vi "OpenEthConnection.vi"(10 "Port":u16=80, 11 "IP address":string="192.168.1.150") -> (0 "error out":errorcluster, 3 "connection ID out":refnum<k5>, 4 "Answer":string="\n\r\n")   [LabVIEW 2015, in "VIPM2.lvlib"]
uses:
  VIPM2.lvlib
panel:
  # "Open Ethernet connection"
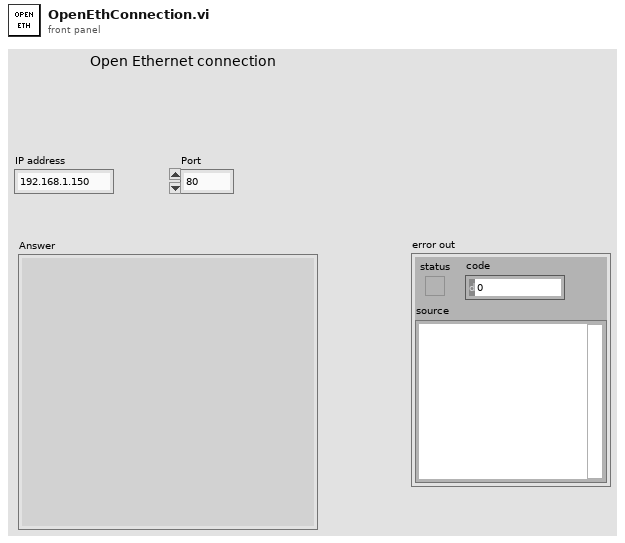
[diagram p1: front panel]
types:
  T1 = enum16{"Standard", "Buffered", "CRLF", "Immediate"}
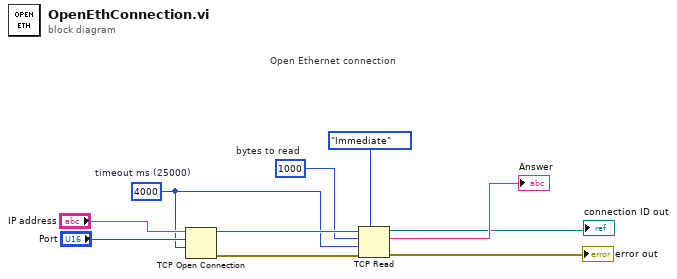
[diagram p0: block diagram]
diagram:
  w3 = 1000  # bytes to read
  w1 = 4000  # timeout ms (25000)
  # "Open Ethernet connection"
  n1 = TCP Open Connection(address="IP address", remote port or service name="Port", timeout ms (60000)=w1) -> (connection ID=w8:refnum<k5>, error out=w7:errorcluster)  [unwired: 2 in]
  n2 = TCP Read(connection ID=w8, bytes to read=w3, error in (no error)=w7, 7:T1."Immediate" ("mode (standard)"), 9:w1) -> (connection ID out=→"connection ID out":refnum<k5>, data out=→"Answer":string, error out=→"error out":errorcluster)
